vi "writeToXML.vi"(8 "error in (no error)":errorcluster, 10 "Class Label":string, 11 "ClockTimes in":refnum<class "ClockTimes.lvclass">) -> (0 "error out":errorcluster, 2 "XML out":string, 3 "ClockTimes out":refnum<class "ClockTimes.lvclass">)   [LabVIEW 2022 SP3, in "TCSDataDefinitions.lvlib" / "TCSPublicStatus.lvlib" / "CurrentTimes.lvlib" / "ClockTimes.lvclass"]
uses:
  ClockTimes.lvclass
  <userlib>/Common/UnitsAndXML/FlattenItemWithUnitToXML/FlattenTimeToXML/TimeUnit.ctl
  ClockTimes.lvclass/ClockTimes.ctl
  <userlib>/Common/UnitsAndXML/UnitsAndXML.lvlib
  <userlib>/Common/XML/XMLGenerator/XMLGenerator.lvclass
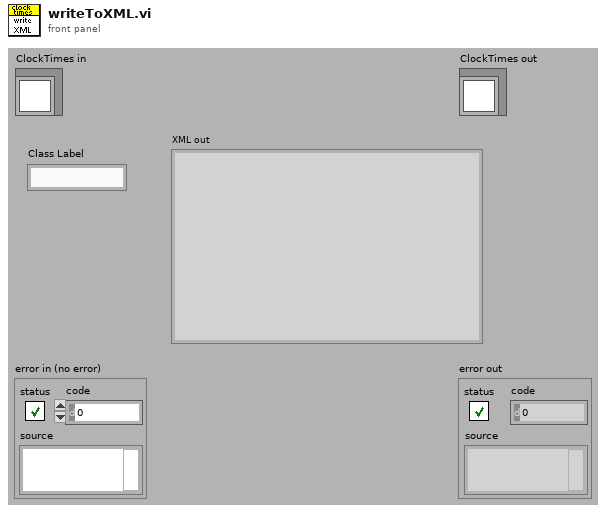
[diagram p1: front panel]
types:
  T1 = typedef "UnitsAndXML.lvlib/TimeUnit.ctl" = enum16{"s", "d", "h", "min", "a"}
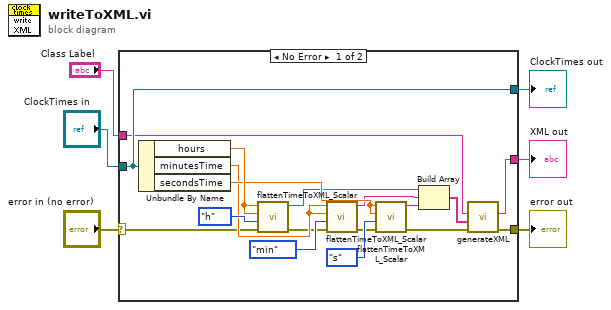
[diagram p0: block diagram]
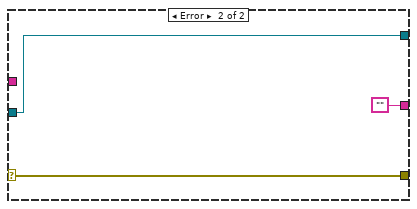
[diagram p2: hidden frame]
diagram:
  n1 = case shown="No Error" "error in (no error)" {
    selector: "error in (no error)" -> [w9 w27]
    tunnel: [w23 w27] -> w5
    tunnel: [w24 w26] -> w4
    tunnel: "ClockTimes in" -> [w24 w26]
    tunnel: [w22 ""] -> w3
    tunnel: "Class Label" -> [w21 _]
    frame No Error {
      n2 = Unbundle By Name(w24) -> ("hours"=w20:dbl[unit], "minutesTime"=w15:dbl[unit], "secondsTime"=w16:dbl[unit])
      n3 = call <userlib>:"flattenTimeToXML_Scalar.vi"("error in (no error)"=w9, "timeUnitInXML"=TimeUnit."h", "timeAgain"=w20, "time"=w20) -> ("error out"=w10:errorcluster, "xmlString"=w14:string)  [unwired: 6 in]
      n4 = call <userlib>:"flattenTimeToXML_Scalar.vi"("error in (no error)"=w10, "timeUnitInXML"=TimeUnit."min", "timeAgain"=w15, "time"=w15) -> ("error out"=w11:errorcluster, "xmlString"=w13:string)  [unwired: 6 in]
      n5 = call <userlib>:"flattenTimeToXML_Scalar.vi"("error in (no error)"=w11, "timeUnitInXML"=TimeUnit."s", "timeAgain"=w16, "time"=w16) -> ("error out"=w8:errorcluster, "xmlString"=w12:string)  [unwired: 6 in]
      n6 = Build Array(w14, w13, w12) -> (w7:string[])
      n7 = call <userlib>:"generateXML.vi"("error in"=w8, "childrenXML"=w7, "elementName"=w21) -> ("error out"=w23:errorcluster, "XML out"=w22:string)  [unwired: 6 in, 1 out]
    }
    frame Error {
    }
  }
  "error out" <- w5
  "ClockTimes out" <- w4
  "XML out" <- w3
